vi "Move Template Files (SubVI).vi"(10 "Template Files Path":path=path "C:/Documents and Settings/lsergent/Desktop/Custom Device Project/Template Files", 11 "Custom Device Folder":path) -> (0 "error out":errorcluster)   [LabVIEW 2010]
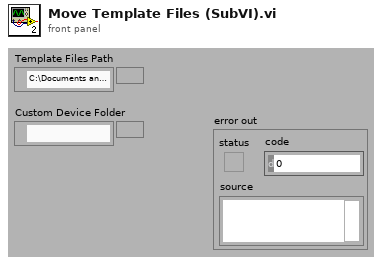
[diagram p1: front panel]
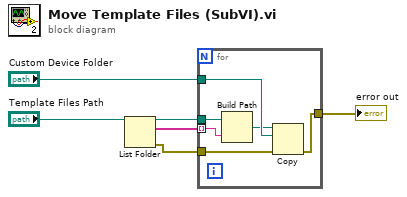
[diagram p0: block diagram]
diagram:
  n1 = List Folder(path="Template Files Path") -> (path out=w4:path, filenames=w3:string[], error out=w5:errorcluster)  [unwired: 3 in, 1 out]
  n2 = for {
    tunnel: "Custom Device Folder" -> [w12]
    tunnel: w3 -> [w11] mode=indexing
    tunnel: w4 -> [w10]
    tunnel: w5 -> [w8]
    tunnel: [w7] -> w2
    n3 = Build Path(base path=w10, name or relative path=w11) -> (appended path=w9:path)
    n4 = Copy(8:w8, 10:w12, 11:w9) -> (0:w7:errorcluster)  [unwired: 2 in, 2 out]
  }
  "error out" <- w2
